vi "8OR.vi"(0 "Boolean":bool, 1 "Boolean 2":bool, 2 "Boolean 3":bool, 3 "Boolean 4":bool, 4 "Boolean 5":bool, 5 "Boolean 6":bool, 6 "Boolean 7":bool, 7 "Boolean 8":bool) -> (23 "Boolean 9":bool)   [LabVIEW 2018]
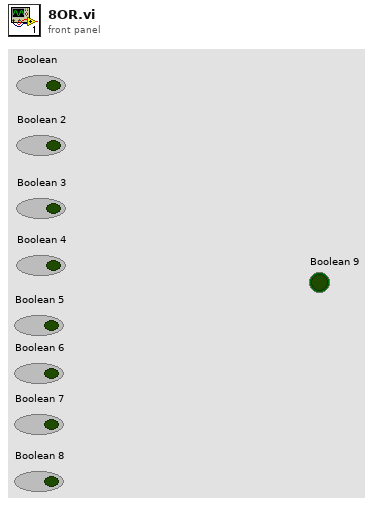
[diagram p1: front panel]
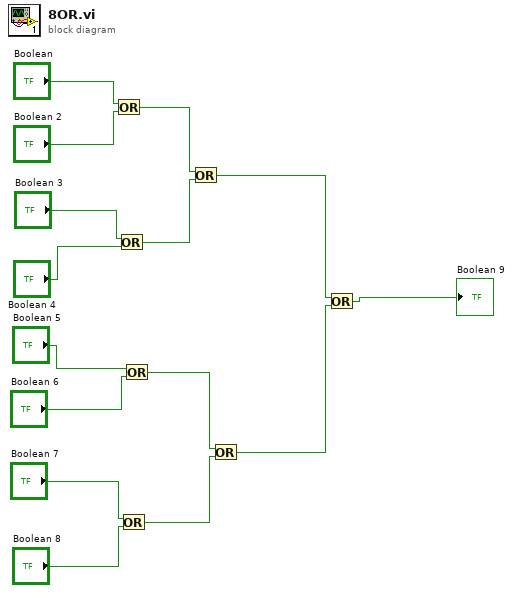
[diagram p0: block diagram]
diagram:
  n1 = Or(x="Boolean", y="Boolean 2") -> (x .or. y?=w6:bool)
  n2 = Or(x="Boolean 3", y="Boolean 4") -> (x .or. y?=w7:bool)
  n3 = Or(x="Boolean 7", y="Boolean 8") -> (x .or. y?=w11:bool)
  n4 = Or(x="Boolean 5", y="Boolean 6") -> (x .or. y?=w10:bool)
  n5 = Or(x=w6, y=w7) -> (x .or. y?=w3:bool)
  n6 = Or(x=w10, y=w11) -> (x .or. y?=w2:bool)
  n7 = Or(x=w3, y=w2) -> (x .or. y?=→"Boolean 9":bool)
